vi "pressure_test.vi"() -> (0 "Gauge":dbl(knob) scale=0.0..10.0)   [LabVIEW 2018]
panel:
  in  "OK Button":bool
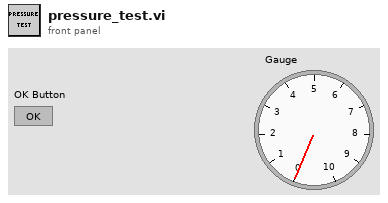
[diagram p1: front panel]
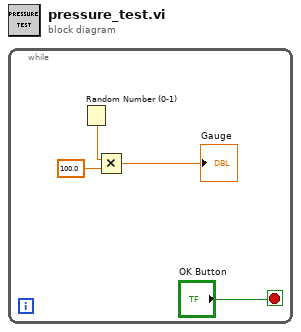
[diagram p0: block diagram]
diagram:
  n1 = while {
    stop <- "OK Button" stop-if-true
    n2 = Random Number (0-1)() -> (number: 0 to 1=w3:dbl)
    n3 = Multiply(x=w3, y=100.0) -> (x*y=→"Gauge":dbl)
  }
